vi "ChannelSettingsQuery.vi"(8 "error in":errorcluster, 11 "T560Channel in":refnum<class "T560Output.lvclass">) -> (0 "error out":errorcluster, 3 "T560Channel out":refnum<class "T560Output.lvclass">)   [LabVIEW 2013, in "T560Output.lvclass"]
doc: "Prepare a command to query the channel settings"
uses:
  T560Output.lvclass
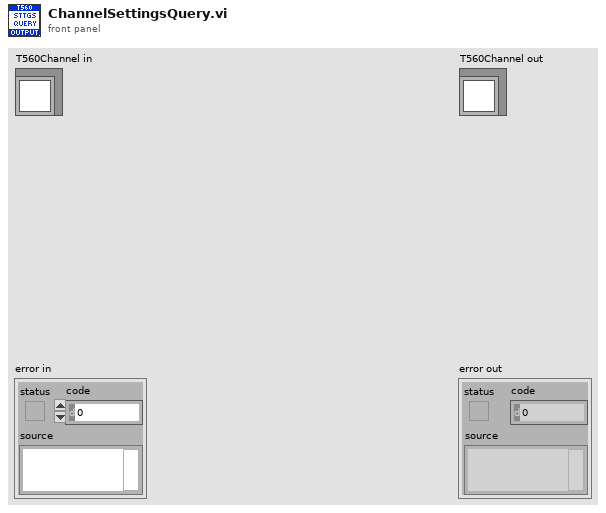
[diagram p1: front panel]
types:
  T1 = typedef "Highlandt564.lvlib/T560Channel.lvclass/ChannelName.ctl" = enum16{"Null", "A", "B", "C", "D", "Trigger"}
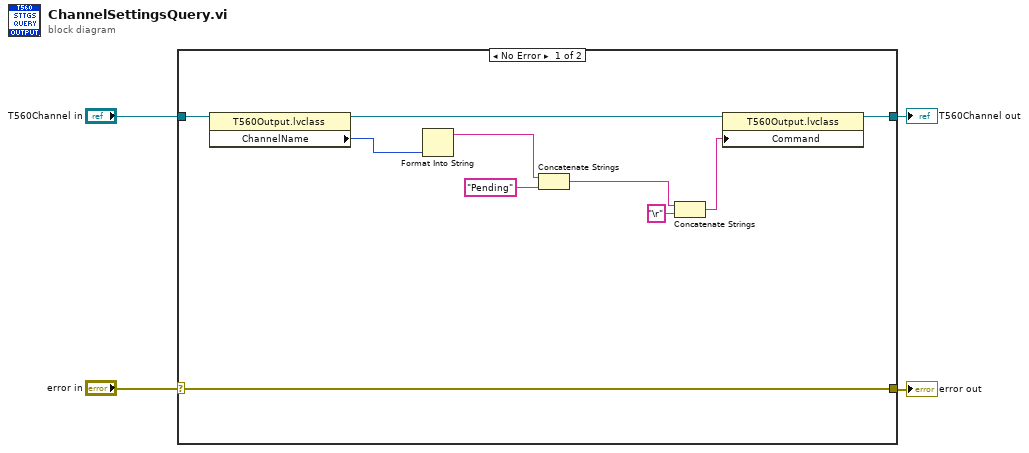
[diagram p0: block diagram]
diagram:
  n1 = case shown="No Error" "error in" {
    selector: "error in" -> [w6 w16]
    tunnel: "T560Channel in" -> [w9 w15]
    tunnel: [w6 w16] -> w4
    tunnel: [w10 w15] -> w3
    frame No Error {
      n2 = property class="T560Output.lvclass"(reference=w9) -> (reference out=w8:refnum<class "T560Output.lvclass">, "ChannelName"=w7:T1)  [unwired: 1 in, 1 out]
      n3 = Format Into String(w7) -> (resulting string=w13:string)  [unwired: 3 in, 1 out]
      n4 = Concatenate Strings(w13, "Pending") -> (w5:string)
      n5 = Concatenate Strings(w5, "\r" ("string")) -> (w11:string)
      n6 = property class="T560Output.lvclass"(reference=w8, "Command"=w11) -> (reference out=w10:refnum<class "T560Output.lvclass">)  [unwired: 1 in, 1 out]
    }
    frame Error {
    }
  }
  "error out" <- w4
  "T560Channel out" <- w3
